vi "Save Current Value Table To Disk.vi"(7 "Force Lookup? (F)":bool, 8 "error in (no error)":errorcluster, 11 "XML File Path":path) -> (0 "error out":errorcluster)   [LabVIEW 2010, in "Current Value Table.lvlib"]
doc: "This VI will save the entire CVT to disk. On the first call, it will produce a list of every tag in the CVT, and fetch the lookup information for each tag. Then, it will retrieve the actual data and format it into a list of tags and save those tags to disk at the path specified. On subsequent calls, unless the (Re)initialize? boolean is set, it will simply store those same tags to disk even if more tags have been added. \nNOTE: This VI is non-reentrant, so this behavior works across multiple instances of this VI."
uses:
  Current Value Table.lvlib
  <vilib>/Utility/xml.llb/Write to XML File(string).vi
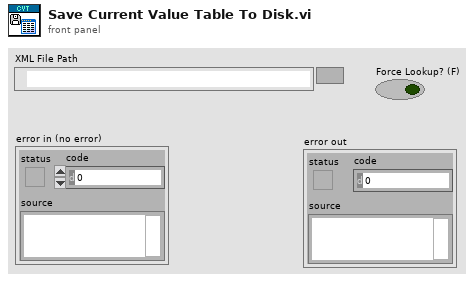
[diagram p1: front panel]
types:
  T1 = typedef "Current Value Table.lvlib/File Format.ctl" = cluster{"Tags":T2[], "Group Listings":T4[]}
  T2 = typedef "Current Value Table.lvlib/Single Tag.ctl" = cluster{"Data Type":T3, "Name":string, "Value":string, "Description":string}
  T3 = typedef "Current Value Table.lvlib/Data Types.ctl" = enum16{"Double", "Single", "I64", "I32", "I16", "I8", "U64", "U32", "U16", "U8", "String", "Boolean", "Array of U8", "Array of U16", "Array of U32", "Array of U64", "Array of I64", "Array of I32", "Array of I16", "Array of I8", "Array of Double", "Array of Single", "Array of Boolean", "Array of String"}
  T4 = typedef "Current Value Table.lvlib/Tag Grouping set.ctl" = cluster{"Group":string, "Tag Names":string[]}
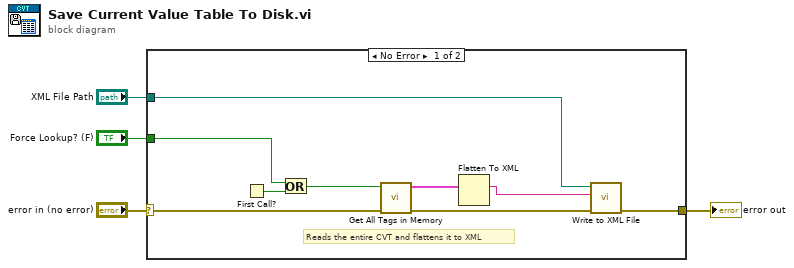
[diagram p0: block diagram]
diagram:
  n1 = case shown="No Error" "error in (no error)" {
    selector: "error in (no error)" -> [w12 w14]
    tunnel: "XML File Path" -> [w8 _]
    tunnel: [w7 w14] -> w2
    tunnel: "Force Lookup? (F)" -> [w5 _]
    frame No Error {
      # "Reads the entire CVT and flattens it to XML"
      n2 = First Call?() -> (First Call?: T/F=w13:bool)
      n3 = Or(x=w5, y=w13) -> (x .or. y?=w11:bool)
      n4 = call "Get All Tags in Memory.vi"("error in (no error)"=w12, "(Re)initialize?"=w11) -> ("error out"=w9:errorcluster, "CVT File Data"=w10:T1)  [unwired: 8 in]
      n5 = Flatten To XML(anything=w10) -> (xml string=w6:string)
      n6 = call-poly <vilib>:"Write to XML File.vi"("error in (no error)"=w9, "XML Input"=w6, "XML File Path"=w8) -> ("error out"=w7:errorcluster)  [unwired: 6 in, 2 out]
    }
    frame Error {
    }
  }
  "error out" <- w2
